vi "Digest Message.vi"(8 "error in (no error)":errorcluster, 10 "MSG":string, 11 "SEQ in":refnum<class "SEQ.lvclass">) -> (0 "error out":errorcluster, 2 "MSG Out":string, 3 "SEQ out":refnum<class "SEQ.lvclass">)   [LabVIEW 2016, in "Sequence Composition.lvlib" / "SEQ.lvclass"]
doc: "Tags the output message with the originating sequence ID and the execution time."
uses:
  SEQ.lvclass
  SEQ.lvclass/SEQ.ctl
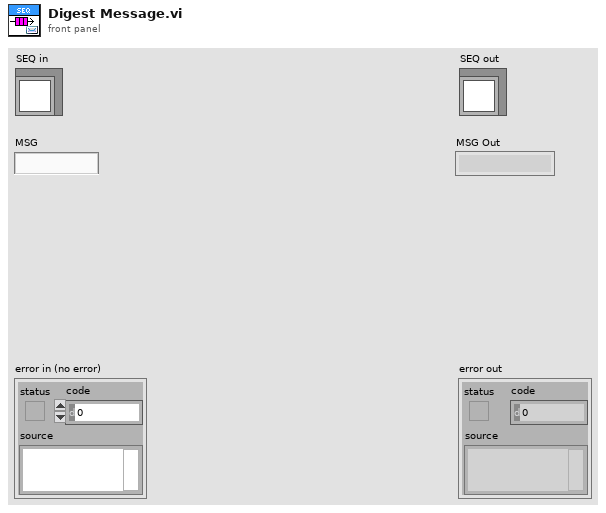
[diagram p1: front panel]
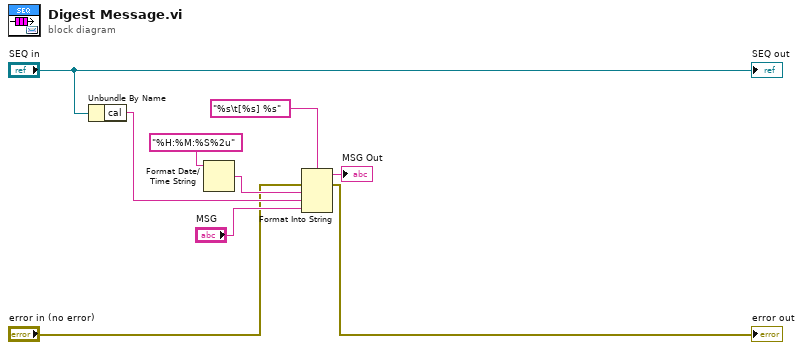
[diagram p0: block diagram]
diagram:
  n1 = Unbundle By Name("SEQ in") -> ("cal"=w5:string)
  n2 = Format Date/Time String(time format string (%c)="%H:%M:%S%2u") -> (date/time string=w6:string)  [unwired: 2 in]
  n3 = Format Into String(format string="%s\t[%s] %s", error in="error in (no error)", w6, w5, "MSG") -> (resulting string=→"MSG Out":string, error out=→"error out":errorcluster)  [unwired: 1 in]
  "SEQ out" <- "SEQ in"
